vi "Flow Setpoint SI.vi"(7 "Set? (F:Read)":bool, 8 "Error In":errorcluster, 9 "Flow Setpoint (0 l/min)":dbl[unit], 10 "Channel (0)":i32, 11 "VISA resource name":refnum<visa-resource-name>) -> (0 "Error Out":errorcluster, 1 "Flow Setpoint out":dbl[unit], 3 "dup VISA resource name":refnum<visa-resource-name>)   [LabVIEW 2016, in "MGC647C.lvlib"]
doc: "Read/Set flow setpoint of a channel in SI unit."
uses:
  MGC647C.lvlib
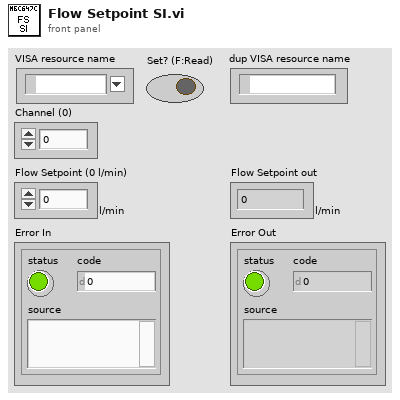
[diagram p1: front panel]
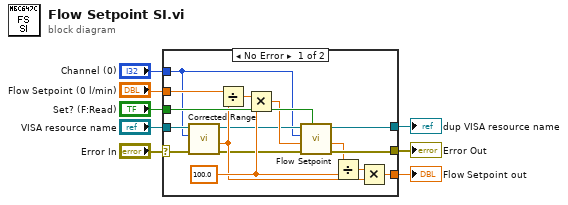
[diagram p0: block diagram]
diagram:
  n1 = case shown="No Error" "Error In" {
    selector: "Error In" -> [w12 w26]
    tunnel: "VISA resource name" -> [w13 w25]
    tunnel: [w23 w25] -> w7
    tunnel: [w22 w26] -> w6
    tunnel: "Set? (F:Read)" -> [w24 _]
    tunnel: "Flow Setpoint (0 l/min)" -> [w16 w27]
    tunnel: [w19 w27] -> w2
    tunnel: "Channel (0)" -> [w9 _]
    frame No Error {
      w15 = 100.0 ("y")
      n2 = call "Corrected Range.vi"("Error In"=w12, "Channel (0)"=w9, "VISA resource name"=w13) -> ("Error Out"=w11:errorcluster, "Corrected Range"=w14:dbl[unit], "dup VISA resource name"=w10:refnum<visa-resource-name>)  [unwired: 6 in]
      n3 = Divide(x=w16, y=w14) -> (x/y=w18:dbl)
      n4 = Multiply(x=w18, y=w15) -> (x*y=w17:dbl)
      n5 = call "Flow Setpoint.vi"("Set? (F:Read)"=w24, "Error In"=w11, "Flow Setpoint (0%)"=w17, "Channel (0)"=w9, "VISA resource name"=w10) -> ("Error Out"=w22:errorcluster, "Flow Setpoint out"=w20:dbl, "dup VISA resource name"=w23:refnum<visa-resource-name>)  [unwired: 4 in]
      n6 = Divide(x=w20, y=w15) -> (x/y=w21:dbl)
      n7 = Multiply(x=w21, y=w14) -> (x*y=w19:dbl[unit])
    }
    frame Error {
    }
  }
  "dup VISA resource name" <- w7
  "Error Out" <- w6
  "Flow Setpoint out" <- w2
